vi "Validate Route.vi"(10 "Path":T1[](array[typedef]), 11 "All Caves":T1[](array[typedef])) -> (2 "End?":bool, 3 "Invalid Path?":bool)   [LabVIEW 2019, in "Day 12.lvlib"]
uses:
  Day 12.lvlib
  Controls/Cave.ctl
  Controls/Cave Type.ctl
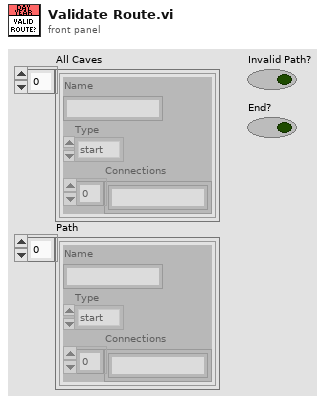
[diagram p1: front panel]
types:
  T1 = typedef "Day 12.lvlib/Cave.ctl" = cluster{"Name":string, "Type":T2, "Connections":string[]}
  T2 = typedef "Day 12.lvlib/Cave Type.ctl" = enum16{"start", "end", "small", "big"}
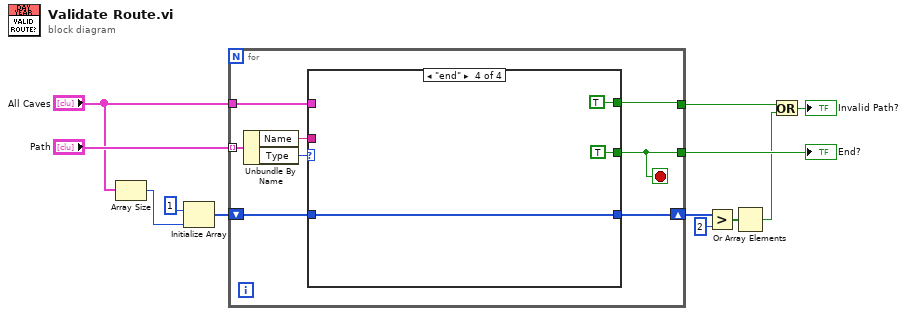
[diagram p0: block diagram]
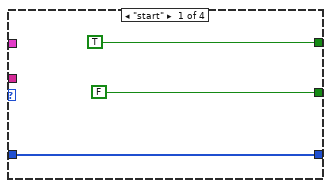
[diagram p2: hidden frame]
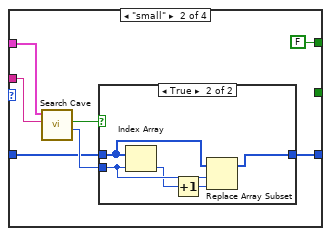
[diagram p3: hidden frame]
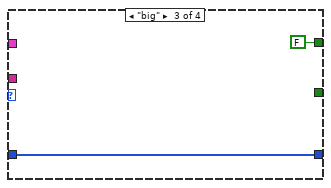
[diagram p5: hidden frame]
diagram:
  n1 = Array Size(array="All Caves") -> (size(s)=w9:i32)
  n2 = Initialize Array(1 ("Cave counter"), w9) -> (w8:i32[])
  n3 = for {
    tunnel: "Path" -> [w20] mode=indexing
    shift-right: [w15] -> w5
    shift-left: w8 -> [w16]
    tunnel: [w18] -> w12
    tunnel: [w17] -> w4
    tunnel: "All Caves" -> [w14]
    stop <- w18 stop-if-true
    n4 = Unbundle By Name(w20) -> ("Name"=w13:string, "Type"=w19:T2)
    n5 = case shown="\"end\"" w19 {
      tunnel: [FALSE _ _ TRUE] -> w18
      tunnel: [TRUE FALSE FALSE TRUE] -> w17
      tunnel: w16 -> [w21 w26 w38 w40]
      tunnel: [w21 w25 w38 w40] -> w15
      tunnel: w14 -> [_ w30 _ _]
      tunnel: w13 -> [_ w29 _ _]
      frame "start" {
      }
      frame "small" {
        n6 = call "Search Cave.vi"("Cave Name"=w29, "Caves"=w30) -> ("Index"=w27:i32, "Found?"=w28:bool)  [unwired: 7 in, 1 out]
        n7 = case shown="True" w28 {
          tunnel: w27 -> [_ w35]
          tunnel: w26 -> [w31 w36]
          tunnel: [w31 w32] -> w25
          frame False {
          }
          frame True {
            n8 = Index Array(array=w36, index=w35) -> (element=w34:i32)
            n9 = Increment(x=w34) -> (x+1=w33:i32)
            n10 = Replace Array Subset(array=w36, new element=w33, index=w35) -> (w32:i32[])
          }
        }
      }
      frame "big" {
      }
      frame "end" {
      }
    }
  }
  "End?" <- w12
  n11 = Greater?(x=w5, y=2) -> (0:w2:bool[])
  n12 = Or Array Elements(Boolean array=w2) -> (logical OR=w1:bool)
  n13 = Or(x=w4, y=w1) -> (x .or. y?=→"Invalid Path?":bool)
